vi "SendNetworkMsg.vi"(0 "reference in":refnum<class "MessageAMC.lvclass">, 1 "receiver process":string, 2 "receiver host":string, 3 "receiver port (0)":u16, 5 "name":string, 7 "value":string, 9 "timeout (25000 ms)":i32=25000, 11 "error in (no error)":errorcluster) -> (4 "reference out":refnum<class "MessageAMC.lvclass">, 10 "timed out?":bool, 15 "error out":errorcluster)   [LabVIEW 2019, in "MessageAMC.lvclass"]
uses:
  MessageAMC.lvclass
  MessageAMC.lvclass/MessageAMC.ctl
  <vilib>/NI/AMC/Create Single Message.vi
  <vilib>/NI/AMC/Update Message Routing Info.vi
  <vilib>/NI/AMC/Send Message.vi
  <vilib>/NI/AMC/AMC.lvlib
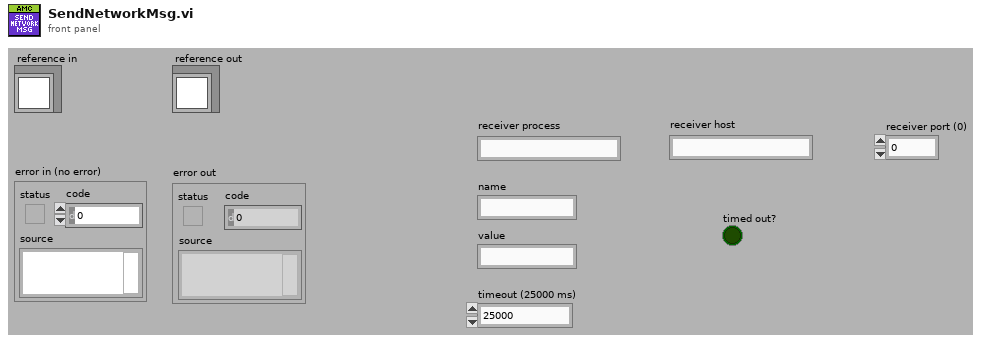
[diagram p1: front panel]
types:
  T1 = typedef "AMC.lvlib/Message Queue.ctl" = refnum<queue>
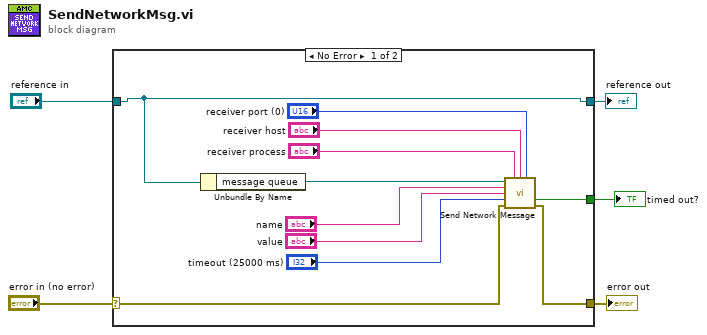
[diagram p0: block diagram]
diagram:
  n1 = case shown="No Error" "error in (no error)" {
    selector: "error in (no error)" -> [w16 w18]
    tunnel: [w9 w18] -> w4
    tunnel: [w6 w17] -> w2
    tunnel: "reference in" -> [w6 w17]
    tunnel: [w8 _] -> w1
    frame No Error {
      n2 = Unbundle By Name(w6) -> ("message queue"=w15:T1)
      n3 = call <vilib>:"Send Network Message.vi"("message queue in"=w15, "receiver process"="receiver process", "receiver host"="receiver host", "receiver port (0)"="receiver port (0)", "message name"="name", "message value"="value", "timeout (25000 ms)"="timeout (25000 ms)", "error in"=w16) -> ("timed out?"=w8:bool, "error out"=w9:errorcluster)  [unwired: 5 in, 1 out]
    }
    frame Error {
    }
  }
  "error out" <- w4
  "reference out" <- w2
  "timed out?" <- w1
